vi "Edit Data Interactively.vi"(8 "error in (no error)":errorcluster, 11 "Data Item in":refnum<class "Data Item.lvclass">) -> (0 "error out":errorcluster, 2 "Cancel?":bool, 3 "Data Item out":refnum<class "Data Item.lvclass">)   [LabVIEW 2023, in "VILab.lvlib" / "Data Item.lvclass"]
uses:
  Data Item.lvclass
  Data Item.lvclass/Data Item.ctl
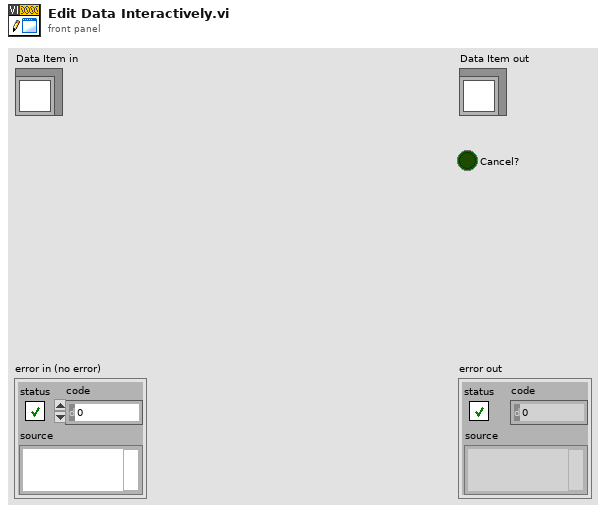
[diagram p1: front panel]
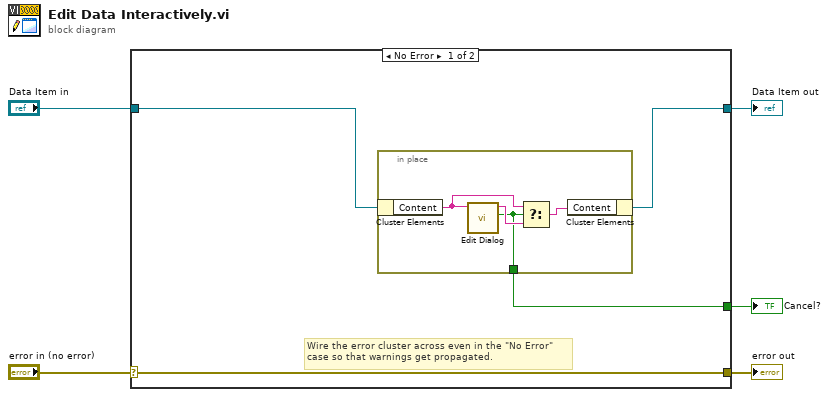
[diagram p0: block diagram]
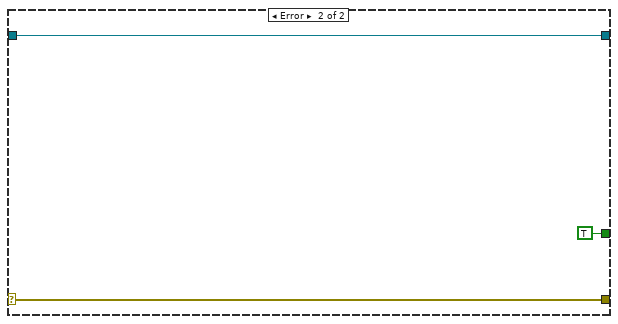
[diagram p2: hidden frame]
diagram:
  n1 = case shown="No Error" "error in (no error)" {
    selector: "error in (no error)" -> [w9 w16]
    tunnel: [w9 w16] -> w4
    tunnel: [w7 w15] -> w2
    tunnel: "Data Item in" -> [w8 w15]
    tunnel: [w6 TRUE ("Canceled?")] -> w1
    frame No Error {
      # "Wire the error cluster across even in the \"No Error\"\ncase so that warnings get propagated."
      n2 = in-place {
        in-place-border: [w10] -> w6
        n3 = in-place-cluster #1(w8) -> ("Content"=w11:string)
        n4 = call "Edit Dialog.vi"("Content"=w11) -> ("Canceled?"=w10:bool, "String"=w13:string)  [unwired: 9 in]
        n5 = Select(t=w11, s=w10, f=w13) -> (s? t:f=w12:string)
        n6 = in-place-cluster #1("Content"=w12) -> (w7:refnum<class "Data Item.lvclass">)
      }
    }
    frame Error {
    }
  }
  "error out" <- w4
  "Data Item out" <- w2
  "Cancel?" <- w1
